vi "CloseActiveSubPanel.vi"(4 "Save?":string, 6 "Create Ref":refnum<vi>, 7 "Mode":string, 8 "error in (no error)":errorcluster, 9 "Modify Ref":refnum<vi>, 10 "close?":refnum<user-event>, 11 "ChannelsRepoBase in":refnum<class "ChannelsRepoXML.lvclass">) -> (0 "error out":errorcluster, 2 "Tag":string, 3 "ChannelsRepoBase out":refnum<class "ChannelsRepoXML.lvclass">)   [LabVIEW 2019]
doc: "Close the active subPanel"
uses:
  ChannelSettingsLib/ChannelsRepos/ChannelsRepoBase/ChannelsRepoBase.lvclass
  ChannelSettingsLib/ChannelsRepos/ChannelsRepoXML/ChannelsRepoXML.lvclass
  C:/Users/DavideAntonoea/Desktop/Repository/channels-setting/source/ChannelSettingsLib/ChannelsRepos/ChannelsRepoBase/ChannelsRepoBase.lvclass
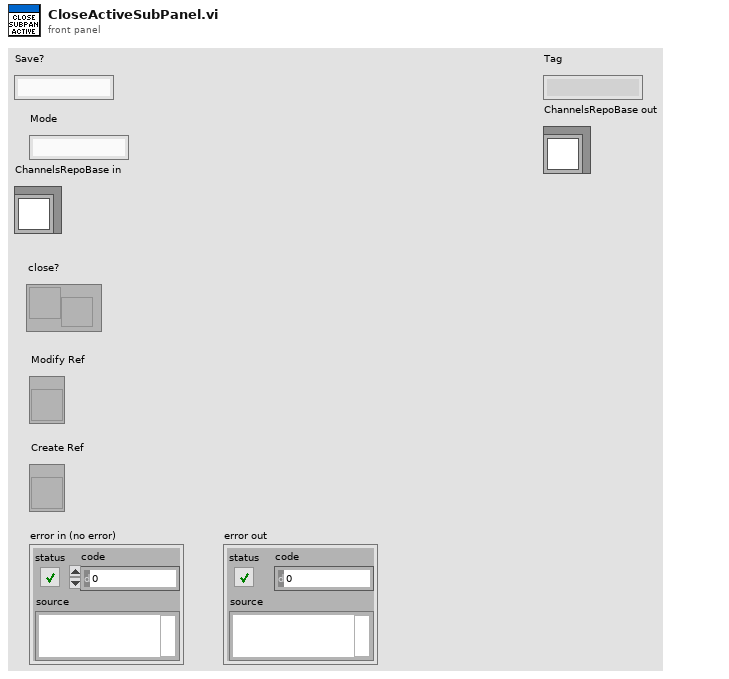
[diagram p1: front panel]
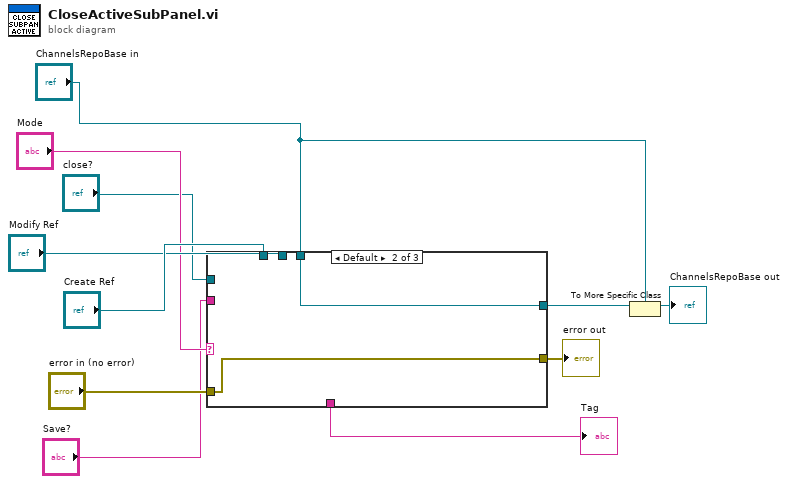
[diagram p0: block diagram]
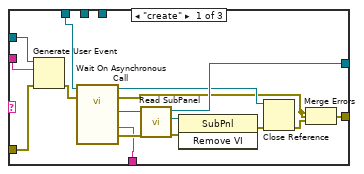
[diagram p2: hidden frame]
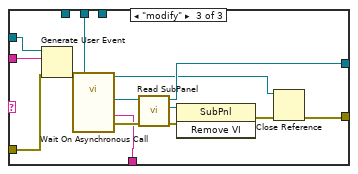
[diagram p3: hidden frame]
diagram:
  n1 = case shown="Default" "Mode" {
    tunnel: [w21 w28 w37] -> w4
    tunnel: [w15 w27 w34] -> w10
    tunnel: "error in (no error)" -> [w18 w27 w33]
    tunnel: "close?" -> [w20 _ w32]
    tunnel: "Modify Ref" -> [_ _ w31]
    tunnel: "ChannelsRepoBase in" -> [_ w28 _]
    tunnel: "Create Ref" -> [w19 _ _]
    tunnel: "Save?" -> [w13 _ w30]
    tunnel: [w12 _ w29] -> w1
    frame "create" {
      n2 = Generate User Event(user event=w20, event data cluster=w13, error in=w18) -> (error out=w23:errorcluster)  [unwired: 1 in, 1 out]
      n3 = call-by-ref "Wait On Asynchronous Call"(reference=w19, error in=w23) -> (reference out=w16:refnum<vi>, error out=w15:errorcluster, 0:"error out"=w22:errorcluster, "Tag"=w12:string, "ChannelBase out"=w24:refnum<class "ChannelsRepoBase.lvclass">)  [unwired: 9 in]
      n4 = call-dynamic "Read SubPanel.vi"("error in (no error)"=w22, "ChannelsRepoBase in"=w24) -> ("error out"=w25:errorcluster, "SubPanel"=w26:refnum<vi>, "ChannelsRepoBase out"=w21:refnum<class "ChannelsRepoBase.lvclass">)  [unwired: 7 in]
      n5 = invoke class="SubPnl" method="Remove VI"(reference=w26, error in=w25) -> (error out=w17:errorcluster)  [unwired: 1 in, 2 out]
      n6 = Close Reference(reference=w16, error in (no error)=w17) -> (error out=w14:errorcluster)
      n7 = Merge Errors(w15, w14) -> ()  [unwired: 1 out]
    }
    frame Default {
    }
    frame "modify" {
      n8 = Generate User Event(user event=w32, event data cluster=w30, error in=w33) -> (error out=w39:errorcluster)  [unwired: 1 in, 1 out]
      n9 = call-by-ref "Wait On Asynchronous Call"(reference=w31, error in=w39) -> (reference out=w35:refnum<vi>, "error out"=w38:errorcluster, "tag"=w29:string, "ChannelsRepoBase out"=w40:refnum<class "ChannelsRepoBase.lvclass">)  [unwired: 9 in, 1 out]
      n10 = call-dynamic "Read SubPanel.vi"("error in (no error)"=w38, "ChannelsRepoBase in"=w40) -> ("error out"=w41:errorcluster, "SubPanel"=w42:refnum<vi>, "ChannelsRepoBase out"=w37:refnum<class "ChannelsRepoBase.lvclass">)  [unwired: 7 in]
      n11 = invoke class="SubPnl" method="Remove VI"(reference=w42, error in=w41) -> (error out=w36:errorcluster)  [unwired: 1 in, 2 out]
      n12 = Close Reference(reference=w35, error in (no error)=w36) -> (error out=w34:errorcluster)
    }
  }
  "error out" <- w10
  "Tag" <- w1
  n13 = To More Specific Class(target class="ChannelsRepoBase in", reference=w4) -> (specific class reference=→"ChannelsRepoBase out":refnum<class "ChannelsRepoXML.lvclass">)  [unwired: 1 in, 1 out]
